vi "EventLoopForStatus.vi"(8 "error in (no error)":errorcluster, 9 "Event Registration Refnum":refnum<event-registration>, 10 "Events":T1, 11 "MulticolumnListbox in":refnum<vi>) -> (0 "error out":errorcluster)   [LabVIEW 2019, in "SolutionBuilder.lvlib"]
uses:
  SolutionBuilder/SolutionBuilder.lvlib
  SolutionBuilder/Events.ctl
  EventUpdateList.ctl
  EventItemBuilt.ctl
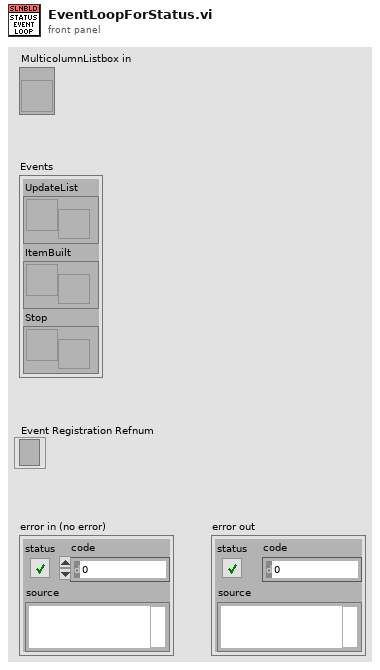
[diagram p1: front panel]
types:
  T1 = typedef "SolutionBuilder.lvlib/Events.ctl" = cluster{"UpdateList":T2, "ItemBuilt":T3, "Stop":refnum<user-event>}
  T2 = typedef "SolutionBuilder.lvlib/EventUpdateList.ctl" = refnum<user-event>
  T3 = typedef "SolutionBuilder.lvlib/EventItemBuilt.ctl" = refnum<user-event>
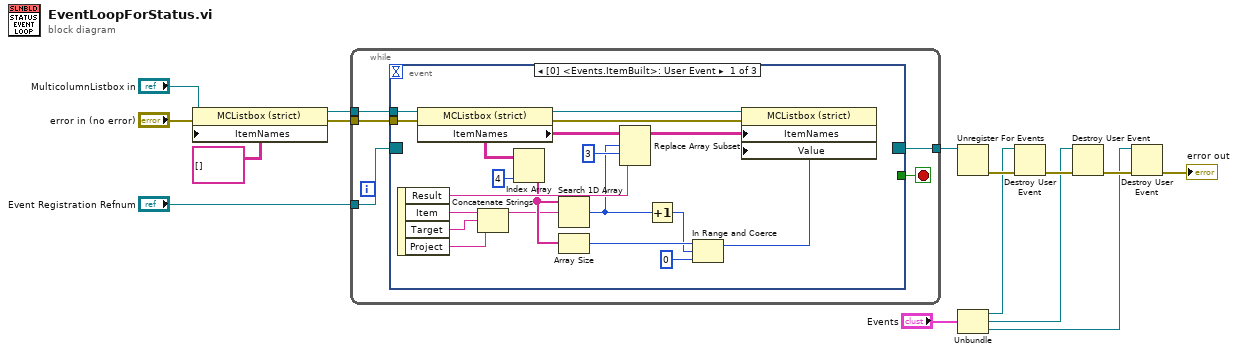
[diagram p0: block diagram]
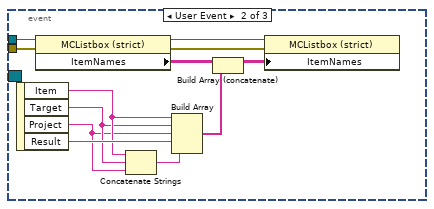
[diagram p2: hidden frame]
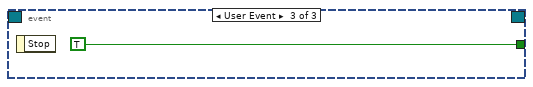
[diagram p3: hidden frame]
diagram:
  n1 = property class="MCListbox (strict)"(reference="MulticolumnListbox in", error in="error in (no error)", "ItemNames"=string[][] [] ("Item Names")) -> (reference out=w7:refnum<vi>, error out=w2:errorcluster)
  n2 = while {
    tunnel: w2 -> [w20]
    tunnel: "Event Registration Refnum" -> [w19]
    tunnel: w7 -> [w17]
    tunnel: [w16] -> w13
    stop <- w18 stop-if-true
    n3 = event shown="[0] <Events.ItemBuilt>: User Event" {
      selector: w19 -> [_ _ _]
      dyn-events: [_ _ _] -> w16
      timeout: _ -> [_ _ _]
      tunnel: w20 -> [w37 w51 _]
      tunnel: [_ _ TRUE] -> w18
      tunnel: w17 -> [w38 w50 _]
      event User Event {
        n4 = event-data() -> ("Result"=w33:string, "Item"=w24:string, "Target"=w23:string, "Project"=w22:string)  [unwired: 1 in]
        n5 = property class="MCListbox (strict)"(reference=w38, error in=w37) -> (reference out=w36:refnum<vi>, error out=w35:errorcluster, "ItemNames"=w32:string[][])
        n6 = Concatenate Strings(w24, w23, w22) -> (w21:string)
        n7 = Index Array(array=w32, index (col)=4 ("disabled index (col)")) -> (element=w29:string[])  [unwired: 1 in]
        n8 = Search 1D Array(1D array=w29, element=w21) -> (index of element=w30:i32)  [unwired: 1 in]
        n9 = Array Size(array=w29) -> (size(s)=w28:i32)
        n10 = Replace Array Subset(array=w32, new element=w33, index (row)=w30, index (col)=3 ("disabled index (col)")) -> (w34:string[][])
        n11 = Increment(x=w30) -> (x+1=w26:i32)
        n12 = In Range and Coerce(upper limit=w28, x=w26, lower limit=0) -> (coerced(x)=w25:i32)  [unwired: 1 out]
        n13 = property class="MCListbox (strict)"(reference=w36, error in=w35, "ItemNames"=w34, "Value"=w25) -> ()  [unwired: 2 out]
      }
      event User Event {
        n14 = event-data() -> ("Item"=w43:string, "Target"=w42:string, "Project"=w41:string, "Result"=w44:string)  [unwired: 1 in]
        n15 = property class="MCListbox (strict)"(reference=w50, error in=w51) -> (reference out=w45:refnum<vi>, error out=w46:errorcluster, "ItemNames"=w49:string[][])
        n16 = Concatenate Strings(w43, w42, w41) -> (w40:string)
        n17 = Build Array(w43, w42, w41, w44, w40) -> (w48:string[])
        n18 = Build Array (concatenate)(w49, w48) -> (w47:string[][])
        n19 = property class="MCListbox (strict)"(reference=w45, error in=w46, "ItemNames"=w47) -> ()  [unwired: 2 out]
      }
      event User Event {
        n20 = event-data() -> ()  [unwired: 1 in, 1 out]
      }
    }
  }
  n21 = Unregister For Events(event registration refnum=w13) -> (error out=w14:errorcluster)  [unwired: 1 in]
  n22 = Unbundle("Events") -> ("UpdateList"=w4:T2, "ItemBuilt"=w3:T3, "Stop"=w5:refnum<user-event>)
  n23 = Destroy User Event(user event=w4, error in=w14) -> (error out=w15:errorcluster)
  n24 = Destroy User Event(user event=w3, error in=w15) -> (error out=w12:errorcluster)
  n25 = Destroy User Event(user event=w5, error in=w12) -> (error out=→"error out":errorcluster)
